vi "Create Continuous Query.vi"(0 "InfluxDB in":refnum<class "Client.lvclass">, 5 "Database name":string, 11 "error in (no error)":errorcluster) -> (4 "InfluxDB out":refnum<class "Client.lvclass">, 15 "error out":errorcluster)   [LabVIEW 2018, in "InfluxDB Client.lvlib" / "Client.lvclass"]
doc: "Creates a database."
uses:
  Client.lvclass
panel:
  in  "Resample duration":i32 format="%<%H:%M:%S>t"
  in  "Resample frequency":i32 format="%<%H:%M:%S>t"
  in  "Query":string
  in  "Continuous query name":string
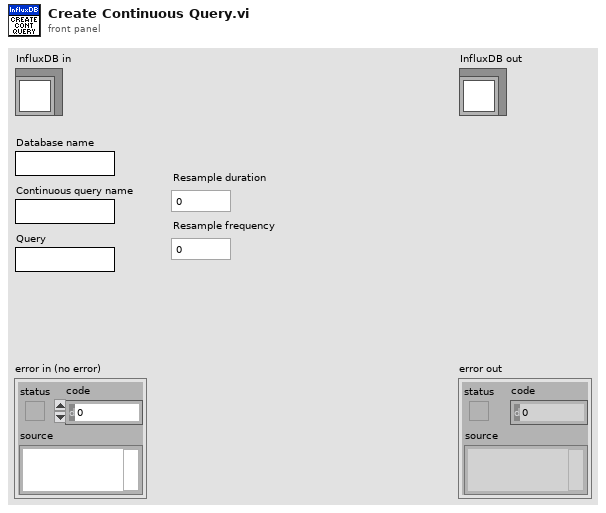
[diagram p1: front panel]
types:
  T1 = typedef "Dictionary Object RefNum__ogtk.ctl" = refnum<k1>
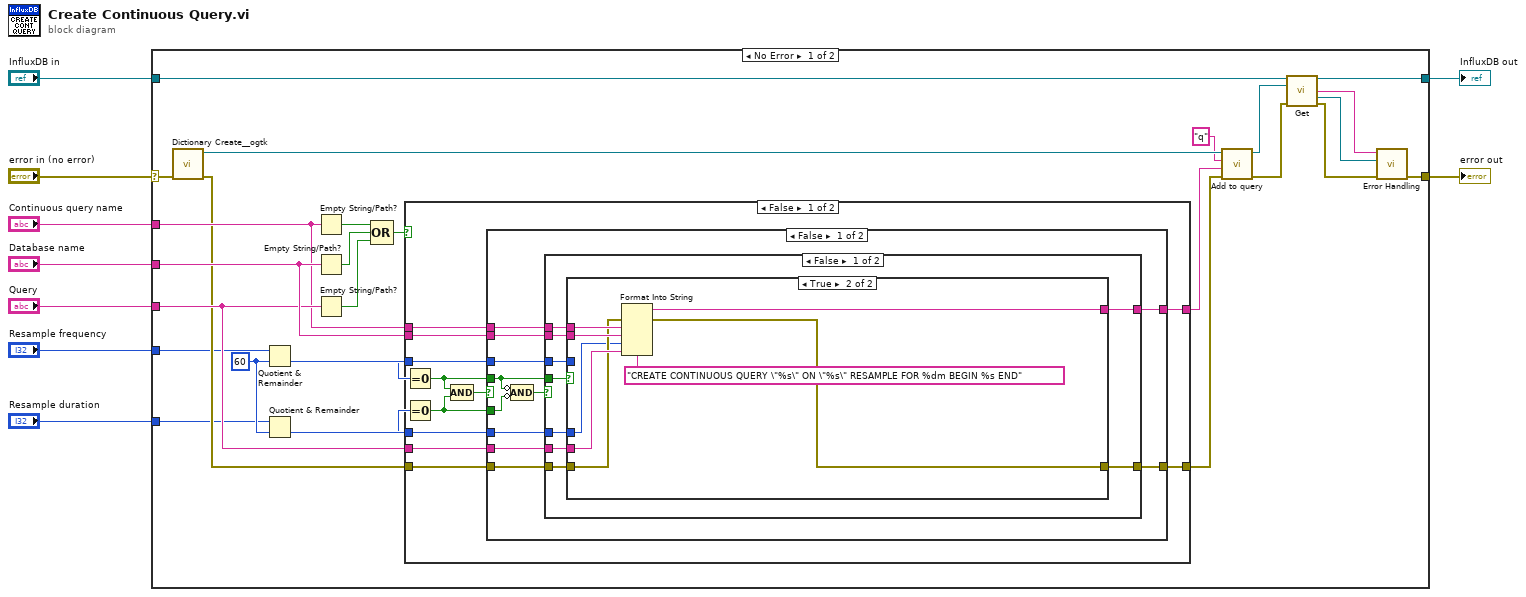
[diagram p0: block diagram]
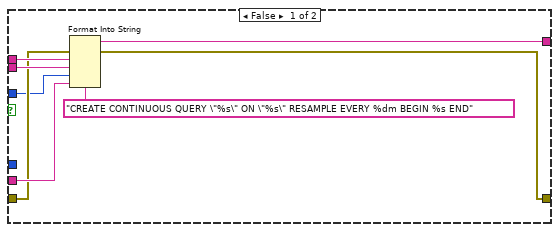
[diagram p2: hidden frame]
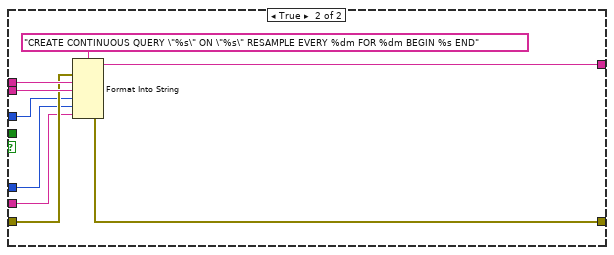
[diagram p3: hidden frame]
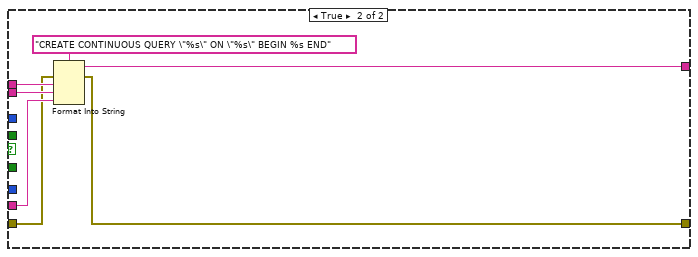
[diagram p4: hidden frame]
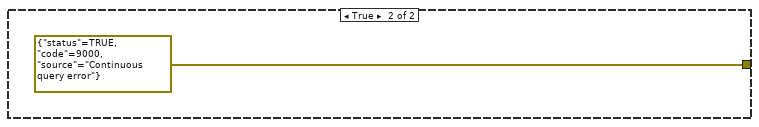
[diagram p5: hidden frame]
diagram:
  n1 = case shown="No Error" "error in (no error)" {
    selector: "error in (no error)" -> [w14 w101]
    tunnel: [w28 w101] -> w9
    tunnel: [w34 w100] -> w7
    tunnel: "InfluxDB in" -> [w35 w100]
    tunnel: "Database name" -> [w18 _]
    tunnel: "Query" -> [w17 _]
    tunnel: "Continuous query name" -> [w16 _]
    tunnel: "Resample frequency" -> [w11 _]
    tunnel: "Resample duration" -> [w10 _]
    frame No Error {
      w19 = 60 ("y")
      n2 = call <userlib>:"Dictionary Create__ogtk.vi"("error in (no error)"=w14) -> ("error out"=w13:errorcluster, "dictionary out"=w33:T1)  [unwired: 9 in]
      n3 = Quotient & Remainder(x=w11, y=w19) -> (floor(x/y)=w24:i32)  [unwired: 1 out]
      n4 = Quotient & Remainder(x=w10, y=w19) -> (floor(x/y)=w25:i32)  [unwired: 1 out]
      n5 = Empty String/Path?(string/path=w16) -> (empty?=w20:bool)
      n6 = Empty String/Path?(string/path=w18) -> (empty?=w21:bool)
      n7 = Empty String/Path?(string/path=w17) -> (empty?=w22:bool)
      n8 = Compound Arithmetic op=OR(w20, w21, w22) -> (w23:bool)
      n9 = case shown="False" w23 {
        tunnel: [w38 errorcluster {"status"=TRUE, "code"=9000, "source"="Continuous query error"} ("error constant")] -> w12
        tunnel: w13 -> [w39 _]
        tunnel: w24 -> [w37 _]
        tunnel: w25 -> [w36 _]
        tunnel: w16 -> [w43 _]
        tunnel: w18 -> [w42 _]
        tunnel: w17 -> [w41 _]
        tunnel: [w40 _] -> w15
        frame False {
          n10 = Equal To 0?(x=w37) -> (x = 0?=w44:bool)
          n11 = Equal To 0?(x=w36) -> (x = 0?=w45:bool)
          n12 = Compound Arithmetic op=AND(w44, w45) -> (w46:bool)
          n13 = case shown="False" w46 {
            tunnel: w45 -> [w57 _]
            tunnel: w44 -> [w55 _]
            tunnel: w43 -> [w54 w97]
            tunnel: w42 -> [w53 w96]
            tunnel: w41 -> [w52 w95]
            tunnel: [w47 w94] -> w40
            tunnel: w39 -> [w51 w93]
            tunnel: [w50 w92] -> w38
            tunnel: w37 -> [w49 _]
            tunnel: w36 -> [w48 _]
            frame False {
              n14 = Compound Arithmetic op=AND(invert w55, invert w57) -> (w56:bool)
              n15 = case shown="False" w56 {
                tunnel: w55 -> [w66 _]
                tunnel: w54 -> [w65 w91]
                tunnel: w53 -> [w64 w90]
                tunnel: w52 -> [w63 w86]
                tunnel: w51 -> [w61 w89]
                tunnel: [w59 w88] -> w50
                tunnel: w49 -> [w62 w85]
                tunnel: w48 -> [w58 w84]
                tunnel: [w60 w83] -> w47
                frame False {
                  n16 = case shown="True" w66 {
                    tunnel: w65 -> [w74 w82]
                    tunnel: w64 -> [w73 w81]
                    tunnel: w63 -> [w72 w80]
                    tunnel: w62 -> [w67 _]
                    tunnel: w61 -> [w71 w79]
                    tunnel: [w69 w77] -> w60
                    tunnel: [w68 w76] -> w59
                    tunnel: w58 -> [_ w75]
                    frame False {
                      n17 = Format Into String(format string="CREATE CONTINUOUS QUERY \"%s\" ON \"%s\" RESAMPLE EVERY %dm BEGIN %s END", error in=w71, w74, w73, w67, w72) -> (resulting string=w69:string, error out=w68:errorcluster)  [unwired: 1 in]
                    }
                    frame True {
                      n18 = Format Into String(format string="CREATE CONTINUOUS QUERY \"%s\" ON \"%s\" RESAMPLE FOR %dm BEGIN %s END", error in=w79, w82, w81, w75, w80) -> (resulting string=w77:string, error out=w76:errorcluster)  [unwired: 1 in]
                    }
                  }
                }
                frame True {
                  n19 = Format Into String(format string="CREATE CONTINUOUS QUERY \"%s\" ON \"%s\" RESAMPLE EVERY %dm FOR %dm BEGIN %s END", error in=w89, w91, w90, w85, w84, w86) -> (resulting string=w83:string, error out=w88:errorcluster)  [unwired: 1 in]
                }
              }
            }
            frame True {
              n20 = Format Into String(format string="CREATE CONTINUOUS QUERY \"%s\" ON \"%s\" BEGIN %s END", error in=w93, w97, w96, w95) -> (resulting string=w94:string, error out=w92:errorcluster)  [unwired: 1 in]
            }
          }
        }
        frame True {
        }
      }
      n21 = call "Add to query.vi"("error in (no error)"=w12, "Value"=w15, "Parameter"="q" ("String"), "Query in"=w33) -> ("error out"=w30:errorcluster, "Query out"=w31:T1)  [unwired: 6 in]
      n22 = call "Get.vi"("InfluxDB Client in"=w35, "Query"=w31, "error in (no error)"=w30) -> ("InfluxDB Client out"=w34:refnum<class "Client.lvclass">, "Status code"=w27:string, "Headers"=w26:T1, "error out"=w29:errorcluster)  [unwired: 8 in, 1 out]
      n23 = call "Error Handling.vi"("error in (no error)"=w29, "HTTP headers"=w26, "HTTP status code"=w27) -> ("error out"=w28:errorcluster)  [unwired: 8 in]
    }
    frame Error {
    }
  }
  "error out" <- w9
  "InfluxDB out" <- w7
